vi "LinearQuadraticRegulator_GetU_Single.vi"(9 "Row":i32, 11 "in LinearQuadraticRegulator":T1) -> (3 "U":dbl)   [LabVIEW 2019, in "Trajectory_Library.lvlib"]
doc: "Returns a single element of the control input vector u.\n \nInputs:\n - LinearQuadraticRegulator -- controller data cluster\n - row -- Index of U to be returned (0-n)\n\nOutputs:\n - U -- The control input single value."
uses:
  Trajectory_Library.lvlib
  TypeDef/LINEAR_QUADRATIC_REGULATOR.ctl
  <vilib>/Analysis/Matrix/Datatypes/RealMatrix.ctl
  <vilib>/Analysis/Matrix/NI_Matrix.lvlib
panel:
  # "Ref State <States,1>"
  # "Comp and capped \noutput <Inputs,1>"
  # "Controller gain\n<Inputs,States>"
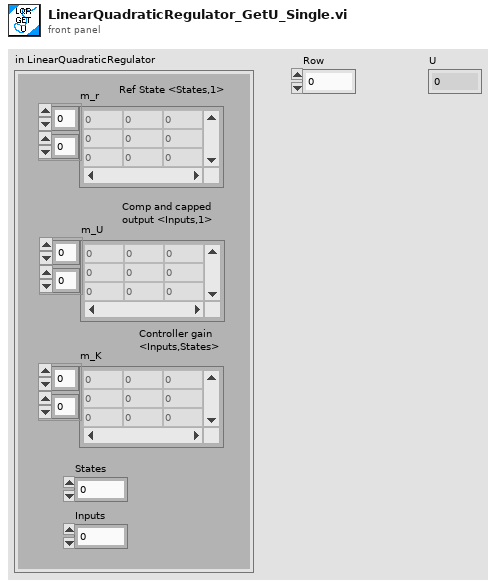
[diagram p1: front panel]
types:
  T1 = typedef "Trajectory_Library.lvlib/LINEAR_QUADRATIC_REGULATOR.ctl" = cluster{"m_r":T2, "m_U":T2, "m_K":T2, "States":i32, "Inputs":i32}
  T2 = typedef "NI_Matrix.lvlib/RealMatrix.ctl" = dbl[][]
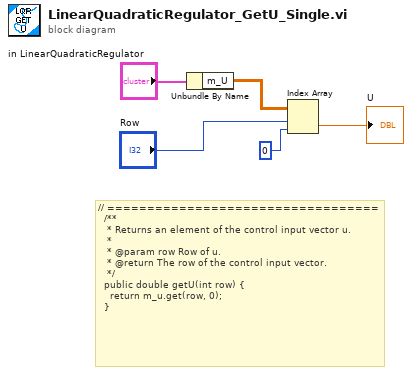
[diagram p0: block diagram]
diagram:
  # "// ==================================\n  /**\n   * Returns an element of the control input vector u.\n   *\n   * @param row Row of u.\n   * @return The row of the control input vector.\n   */\n  public double getU(int row) {\n    return m_u.get(row, 0);\n  }"
  n1 = Unbundle By Name("in LinearQuadraticRegulator") -> ("m_U"=w4:T2)
  n2 = Index Array(array=w4, index (row)="Row", index (col)=0) -> (element=→"U":dbl)
